vi "Scan Multi Bias (With Setpoint Control-REVISED).vi"(0 "Series Name":string="ScanMultiBias_" caption="Serie name", 1 "Avoid zero threshold (V)":dbl=0.004999999888241291 format="%#_13g", 5 "Number of scans":u8=5, 12 "Auto save":bool=TRUE) -> (15 "Error out":errorcluster)   [LabVIEW 2026]
doc: "This example performs multiple image scans, increasing the bias voltage after each scan.\n\n- Nanonis Programming Interface -"
uses:
  <userlib>/Nanonis Prog Interface V5e/Nanonis Prog Interface.lvlib
panel:
  in  "Machine name (local machine IP)":string
  # "Example program for the Nanonis SPM Control software programming interface\n(see diagram)."
  # "SET ALL PARAMETERS FOR # OF SCAN (I.E. 50 scans = 50 Parameters"
  # "This example performs multiple image scans, increasing the bias voltage after each scan."
  # "Change Bias based on iteration of scan"
  # "Change Setpoint based on iteration of scan"
  # "Set to 0.05M to go from -100 mV to 100 mV"
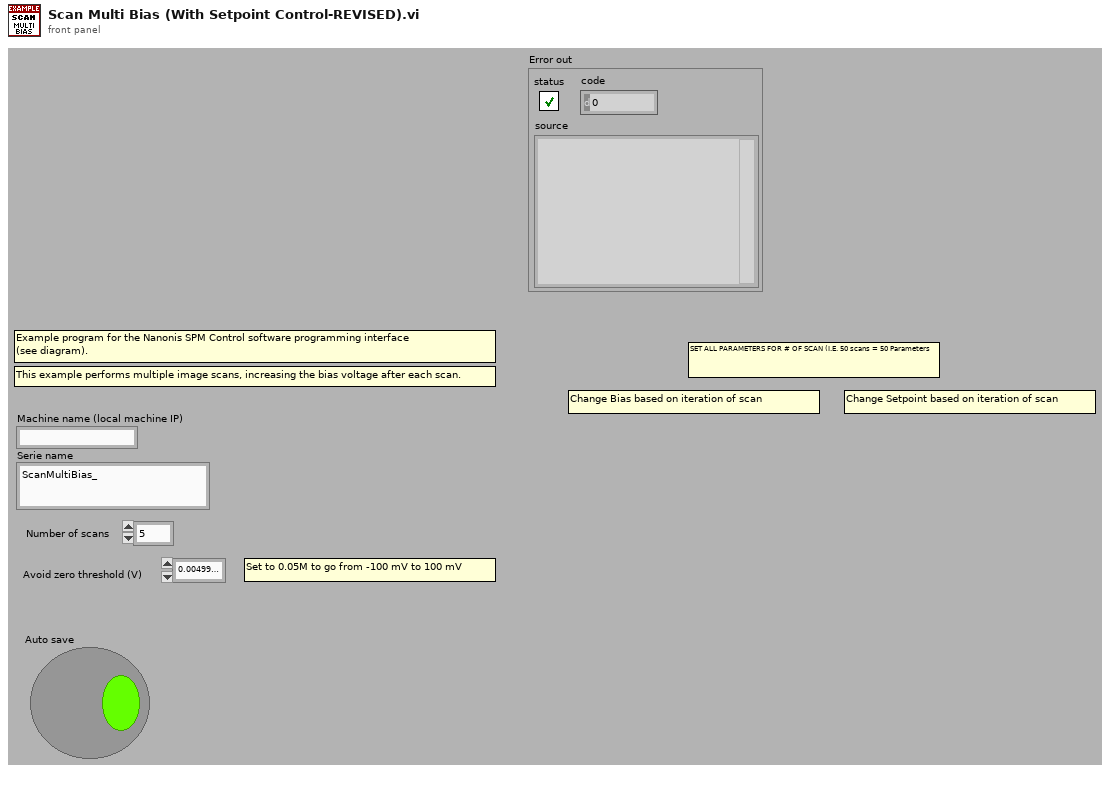
[diagram p1: front panel]
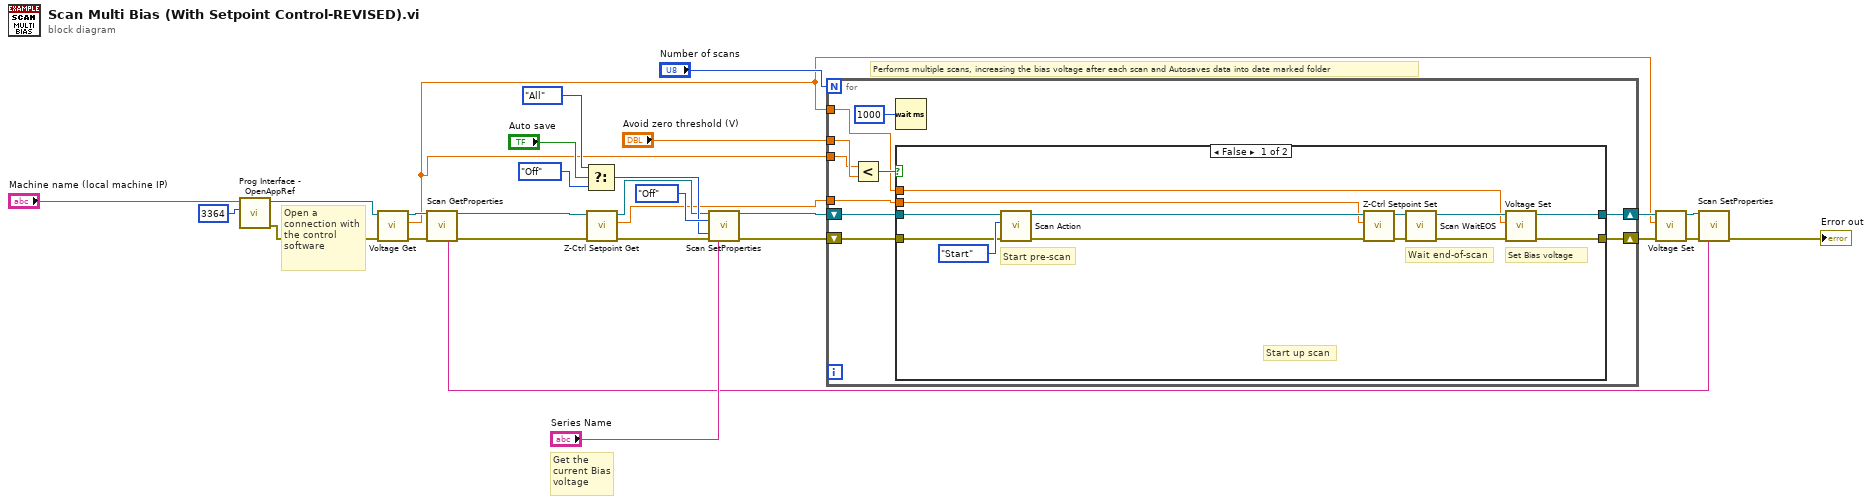
[diagram p0: block diagram]
diagram:
  # "Open a connection with the control\nsoftware"
  # "Performs multiple scans, increasing the bias voltage after each scan and Autosaves data into date marked folder"
  # "Get the current Bias voltage"
  n1 = call <userlib>:"Prog Interface - OpenAppRef.vi"("Port number (3364)"=u32 3364, "Machine name (local machine IP)"="Machine name (local machine IP)") -> ("Error out"=w28:errorcluster, "Application reference"=w20:refnum<vi>)  [unwired: 4 in]
  n2 = call <userlib>:"Voltage Get.vi"("error in (no error)"=w28, "Application ref in"=w20) -> ("error out"=w15:errorcluster, "Bias (V)"=w1:sgl, "Application ref out"=w16:refnum<vi>)  [unwired: 7 in]
  n3 = call <userlib>:"Scan GetProperties.vi"("Application ref in"=w16, "Error in (no error)"=w15) -> ("Application ref out"=w11:refnum<vi>, "Serie name"=w14:string, "Error out"=w12:errorcluster)  [unwired: 5 in, 6 out]
  n4 = Select(t=enum16{"No change", "All", "Next", "Off"}."All" ("Auto save"), s="Auto save", f=enum16{"No change", "All", "Next", "Off"}."Off" ("Auto save")) -> (s? t:f=w21:enum16{"No change", "All", "Next", "Off"})
  n5 = call <userlib>:"Z-Ctrl Setpoint Get.vi"("error in (no error)"=w12, "Application ref in"=w11) -> ("error out"=w9:errorcluster, "Z Controller setpoint"=w2:sgl, "Application ref out"=w10:refnum<vi>)  [unwired: 6 in]
  n6 = call <userlib>:"Scan SetProperties.vi"("Application ref in"=w10, "Continuous scan"=enum16{"No change", "On", "Off"}."Off", "Auto save"=w21, "Error in (no error)"=w9, "Serie name"="Series Name") -> ("Application ref out"=w19:refnum<vi>, "Error out"=w27:errorcluster)  [unwired: 9 in]
  n7 = for {
    N: "Number of scans" -> [_]
    shift-right: [w34] -> w17
    shift-left: w27 -> [w38]
    shift-right: [w35] -> w18
    shift-left: w19 -> [w37]
    tunnel: "Avoid zero threshold (V)" -> [w33]
    tunnel: w1 -> [w31]
    tunnel: w2 -> [w30]
    tunnel: w1 -> [w29]
    n8 = Less?(x=w29, y=w33) -> (x < y?=w36:bool)
    n9 = Wait (ms)(milliseconds to wait=u32 1000) -> ()  [unwired: 1 out]
    n10 = case shown="False" w36 {
      tunnel: w38 -> [w39 w52]
      tunnel: w37 -> [w40 w53]
      tunnel: [w50 w53] -> w35
      tunnel: [w49 w52] -> w34
      tunnel: w31 -> [w42 _]
      tunnel: w30 -> [w41 _]
      frame False {
        # "Start up scan"
        # "Set Bias voltage"
        # "Wait end-of-scan"
        # "Start pre-scan"
        n11 = call <userlib>:"Scan Action.vi"("error in (no error)"=w39, "Scan action (Start)"=enum16{"Start", "Stop", "Pause", "Resume"}."Start" ("Scan action"), "Application ref in"=w40) -> ("error out"=w48:errorcluster, "Application ref out"=w45:refnum<vi>)  [unwired: 6 in]
        n12 = call <userlib>:"Z-Ctrl Setpoint Set.vi"("error in (no error)"=w48, "Z Controller setpoint"=w41, "Application ref in"=w45) -> ("error out"=w47:errorcluster, "Application ref out"=w46:refnum<vi>)  [unwired: 7 in]
        n13 = call <userlib>:"Scan WaitEOS.vi"("error in (no error)"=w47, "Application ref in"=w46) -> ("error out"=w43:errorcluster, "Application ref out"=w44:refnum<vi>)  [unwired: 5 in, 2 out]
        n14 = call <userlib>:"Voltage Set.vi"("Error in (no error)"=w43, "Bias (V)"=w42, "Application ref in"=w44) -> ("Error out"=w49:errorcluster, "Application ref out"=w50:refnum<vi>)  [unwired: 7 in]
      }
      frame True {
      }
    }
  }
  n15 = call <userlib>:"Voltage Set.vi"("Error in (no error)"=w17, "Bias (V)"=w1, "Application ref in"=w18) -> ("Error out"=w7:errorcluster, "Application ref out"=w6:refnum<vi>)  [unwired: 7 in]
  n16 = call <userlib>:"Scan SetProperties.vi"("Application ref in"=w6, "Error in (no error)"=w7, "Serie name"=w14) -> ("Error out"=→"Error out":errorcluster)  [unwired: 11 in, 1 out]
